vi "LV9_3.vi"() -> ()   [LabVIEW 2016]
uses:
  <vilib>/imath/engines/lvmath2/RunTimeEngine/BuiltInFunctions/length/NIMS_length(GV).vi
  <instcachedir>/0/NIMS_length(GV)_08A3D13377FD4E4B96F5795FBF3698FA.lvgen/NIMS_length(GV)_08A3D13377FD4E4B96F5795FBF3698FA_000.vi
  <vilib>/imath/engines/lvmath2/RunTimeEngine/RangeToken/NIMS_Range.vi
  <instcachedir>/0/NIMS_Range_A7C094595B484CA7AF10685B02D808ED.lvgen/NIMS_Range_A7C094595B484CA7AF10685B02D808ED_000.vi
  <vilib>/imath/engines/lvmath2/RunTimeSupport/NIMS_Error if Not Equal.vi
  <instcachedir>/0/NIMS_Error if Not Equal_43252A79AD05436189442EC0C5E5AB8A.lvgen/NIMS_Error if Not Equal_43252A79AD05436189442EC0C5E5AB8A_001.vi
  <vilib>/imath/engines/lvmath2/RunTimeEngine/IndexRead/NIMS V(V).vi
  <instcachedir>/0/NIMS V(V)_298D9CB7BFEB42B8BC8D9C3C28AE8C70.lvgen/NIMS V(V)_298D9CB7BFEB42B8BC8D9C3C28AE8C70_001.vi
  <vilib>/imath/engines/lvmath2/RunTimeEngine/ErrorHandling/NIMS_Create Error From Enums.vi
  <vilib>/imath/engines/lvmath2/RunTimeEngine/BuiltInFunctions/reshapemx/NIMS_[GM]_reshapemx.vi
  <instcachedir>/0/NIMS_[GM]_reshapemx_500BD31B48F5434EA23B2056DCB44201.lvgen/NIMS_[GM]_reshapemx_500BD31B48F5434EA23B2056DCB44201_000.vi
  <vilib>/imath/engines/lvmath2/RunTimeEngine/BuiltInFunctions/fft/NIMS_fft(GM).vi
  <instcachedir>/0/NIMS_fft(GM)_7BD4D6367ED64442B25130C0D1EFC54B.lvgen/NIMS_fft(GM)_7BD4D6367ED64442B25130C0D1EFC54B_000.vi
  <vilib>/imath/engines/lvmath2/RunTimeEngine/BuiltInFunctions/abs/NIMS_abs(signed).vi
  <instcachedir>/0/NIMS_abs(signed)_C4FCB8E6058B49B797C7C8D53CA5F6EC.lvgen/NIMS_abs(signed)_C4FCB8E6058B49B797C7C8D53CA5F6EC_003.vi
  <vilib>/imath/engines/lvmath2/RunTimeEngine/IndexRead/NIMS M(V,$).vi
  <instcachedir>/0/NIMS M(V,$)_21A5155762F74C04AE4EA67BEE0D3EF5.lvgen/NIMS M(V,$)_21A5155762F74C04AE4EA67BEE0D3EF5_004.vi
  <vilib>/imath/engines/lvmath2/RunTimeEngine/BuiltInFunctions/size/NIMS_I32=size(GM,I32).vi
  <instcachedir>/0/NIMS_I32=size(GM,I32)_122058B1B3294FAEA5DC209B92B394E4.lvgen/NIMS_I32=size(GM,I32)_122058B1B3294FAEA5DC209B92B394E4_004.vi
  <vilib>/imathl/engines/lvmath/Functions/Error Handling/Create Error.vi
  <vilib>/imath/engines/lvmath2/RunTimeEngine/NodeEndStatement/NIMS_NodeEndStatement_Output.vi
  <instcachedir>/0/NIMS_NodeEndStatement_Output_53EC0D466D134D7ABD903AC30B43404B.lvgen/NIMS_NodeEndStatement_Output_53EC0D466D134D7ABD903AC30B43404B_005.vi
  <instcachedir>/0/NIMS_NodeEndStatement_Output_53EC0D466D134D7ABD903AC30B43404B.lvgen/NIMS_NodeEndStatement_Output_53EC0D466D134D7ABD903AC30B43404B_010.vi
  <instcachedir>/0/NIMS_NodeEndStatement_Output_53EC0D466D134D7ABD903AC30B43404B.lvgen/NIMS_NodeEndStatement_Output_53EC0D466D134D7ABD903AC30B43404B_002.vi
  <vilib>/imath/engines/lvmath2/RunTimeEngine/ErrorHandling/NIMS_Finalize Error.vi
  <vilib>/picture/picture.llb/Draw 8-Bit Pixmap.vi
panel:
  in  "Spectrogram segments":i32(slide) scale=16.0..64.0
  in  "Stop Button":bool
  in  "Chirp slope":dbl(slide) scale=0.5..1.5
  out "Chirp signal":cluster{"t":dbl[], "X":dbl[]}(graph)
  out "new picture":picture
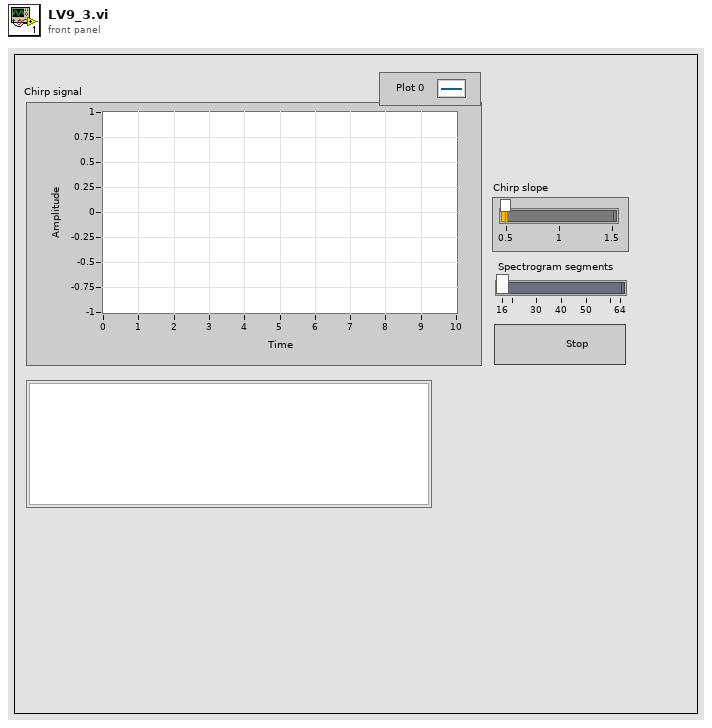
[diagram p1: front panel]
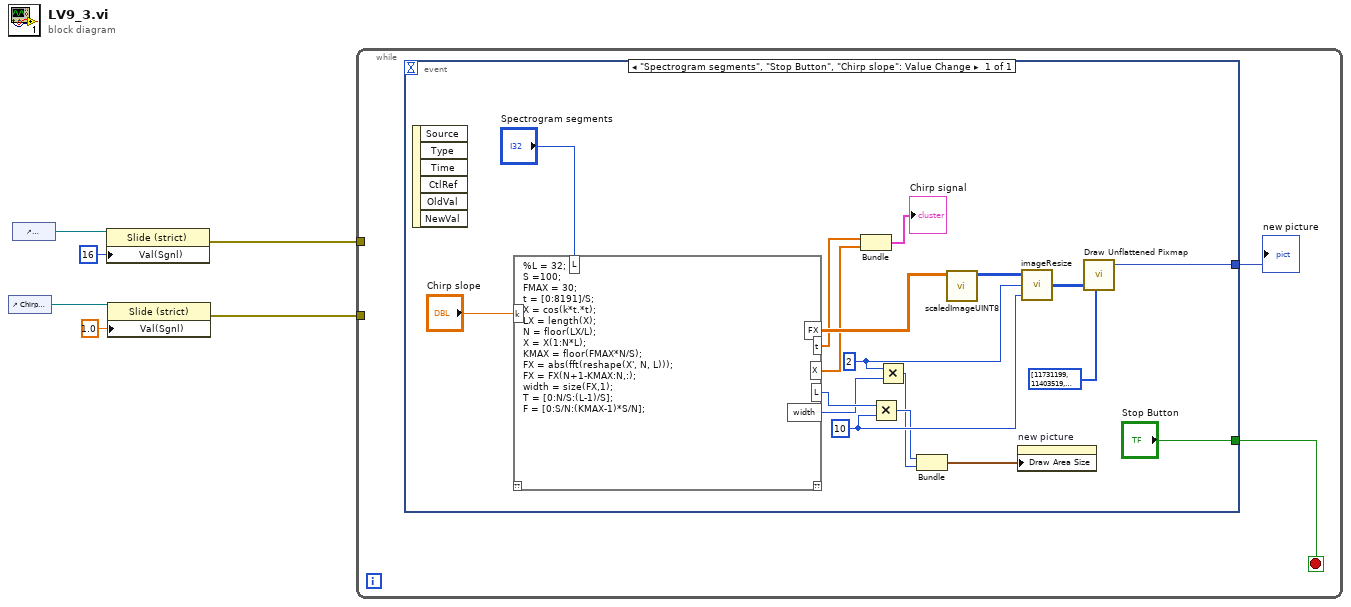
[diagram p0: block diagram]
diagram:
  n1 = control-ref of="Chirp slope"() -> (w4:refnum<vi>)
  n2 = control-ref of="Spectrogram segments"() -> (w1:refnum<vi>)
  n3 = property class="Slide (strict)"(reference=w1, "Val(Sgnl)"=u16 16 ("Value")) -> (error out=w5:errorcluster)  [unwired: 1 in, 1 out]
  n4 = property class="Slide (strict)"(reference=w4, "Val(Sgnl)"=1.0 ("Value")) -> (error out=w2:errorcluster)  [unwired: 1 in, 1 out]
  n5 = while {
    tunnel: w5 -> [_]
    tunnel: w2 -> [_]
    stop <- w7 stop-if-true
    n6 = event shown="[0] \"Spectrogram segments\", \"Stop Button\", \"Chirp slope\": Value Change" {
      selector: _ -> [_]
      dyn-events: _ -> [_]
      timeout: _ -> [_]
      tunnel: [w24] -> w8
      tunnel: ["Stop Button"] -> w7
      event "Spectrogram segments", "Stop Button", "Chirp slope": Value Change {
        w20 = 10 ("factor")
        w21 = 2 ("factor")
        n7 = event-data() -> ()  [unwired: 1 in, 6 out]
        n8 = mathscript code="%L = 32;\nS =100;\nFMAX = 30;\nt = [0:8191]/S;\nX = cos(k*t.*t);\nLX = length(X);\nN = floor(LX/L);\nX = X(1:N*L);\nKMAX = floor(FMAX*N/S);\nFX = abs(fft(reshape(X', N, L)));\nFX = FX(N+1-KMAX:N,:);\nwidth = size(FX,1);\nT = [0:N/S:(L-1)/S];\nF = [0:S/N:(KMAX-1)*S/N];"("k"="Chirp slope", "L"="Spectrogram segments") -> ("FX"=w22:dbl[][], "X"=w13:dbl[], "L"=w18:i32, "width"=w17:i32, "t"=w14:dbl[])  [unwired: 1 in, 1 out]
        n9 = Bundle("t"=w14, "X"=w13) -> (→"Chirp signal":cluster{"t":dbl[], "X":dbl[]})  [unwired: 1 in]
        n10 = Multiply(x=w18, y=w20) -> (x*y=w16:i32)
        n11 = Multiply(x=w21, y=w17) -> (x*y=w15:i32)
        n12 = Bundle(w16, w15) -> (w19:cluster{i32, i32})  [unwired: 1 in]
        n13 = call "scaledImageUINT8.vi"("double image"=w22) -> ("uint8 image"=w25:u8[][])  [unwired: 10 in]
        n14 = property on="new picture" class="Pict"("Draw Area Size"=w19) -> ()  [unwired: 2 in, 2 out]
        n15 = call "imageResize.vi"("colScale"=w20, "rowScale"=w21, "image"=w25) -> ("resized image"=w26:u8[][])  [unwired: 1 in]
        n16 = call-poly <vilib>:"Draw Unflattened Pixmap.vi"("data"=w26, "color table"=u32[] [11731199, 11403519, 11141375, 10813695, 10551551, 10223871, 9961727, 9699583, 9371903, 9109759, 8782079, 8519935, 8257791, 7930111, 7667967, 7405823, 7078143, 6815999, 6488319, 6226175, 5898495, 5636351, 5374207, 5046527, 4784383, 4456703, 4194559, 3932415, 3604735, 3342591, 3014911, 2752767, 2490623, 2162943, 1900799, 1573119, 1310975, 1048831, 721151, 459007, 131327, 767, 1791, 3071, 4095, 5375, 6399, 7423, 8703, 9727, 11007, 12031, 13055, 14335, 15359, 16639, 17663, 18687, 19967, 20991, 22271, 23295, 24319, 25599, 26623, 27903, 28927, 29951, 31231, 32255, 33535, 34559, 35583, 36863, 37887, 39167, 40191, 41215, 42495, 43519, 44799, 45823, 46847, 48127, 49151, 50431, 51455, 52479, 53759, 54783, 56063, 57087, 58111, 59391, 60415, 61695, 62719, 63743, 65023, 65533, 65528, 65524, 65520, 65515, 65511, 65506, 65502, 65498, 65493, 65489, 65484, 65480, 65476, 65471, 65467, 65462, 65458, 65454, 65449, 65445, 65440, 65436, 65432, 65427, 65423, 65418, 65414, 65410, 65405, 65401, 65396, 65392, 65388, 65383, 65379, 65374, 65370, 65366, 65361, 65357, 65352, 65348, 65344, 65339, 65335, 65330, 65326, 65322, 65317, 65313, 65309, 65304, 65300, 65295, 65291, 65286, 65282, 196352, 524032, 786176, 1113856, 1376000, 1638144, 1965824, 2227968, 2555648, 2817792, 3079936, 3407616, 3669760, 3997440, 4259584, 4521728, 4849408, 5111552, 5439232, 5701376, 5963520, 6291200, 6553344, 6881024, 7143168, 7405312, 7732992, 7995136, 8322816, 8584960, 8847104, 9174784, 9436928, 9764608, 10026752, 10288896, 10616576, 10878720, 11206400, 11468544, 11730688, 12058368, 12320512, 12648192, 12910336, 13172480, 13500160, 13762304, 14089984, 14352128, 14614272, 14941952, 15204096, 15531776, 15793920, 16056064, 16383744, 16645888, 16776192, 16775168, 16774144, 16772864, 16771840, 16770560, 16769536, 16768512, 16767232, 16766208, 16764928, 16763904, 16762880, 16761600, 16760576, 16759296, 16758272, 16757248, 16755968, 16754944, 16753664, 16752640, 16751616, 16750336, 16749312, 16748032, 16747008, 16745984, 16744704, 16743680, 16742400, 16741376, 16740352, 16739072, 16738048, 16736768, 16735744, 16734720, 16733440, 16732416, 16731136] ("Array 2")) -> ("new picture"=w24:picture)  [unwired: 7 in]
      }
    }
    "new picture" <- w8
  }
